vi "GetVolume.vi"(0 "reference in":refnum<class "MusicDevice.lvclass">, 5 "Error In":errorcluster) -> (14 "reference out":refnum<class "MusicDevice.lvclass">, 16 "Volume":u8 max=100, 19 "Error Out":errorcluster)   [LabVIEW 2024, in "MusicDevice.lvclass"]
uses:
  MusicDevice.lvclass
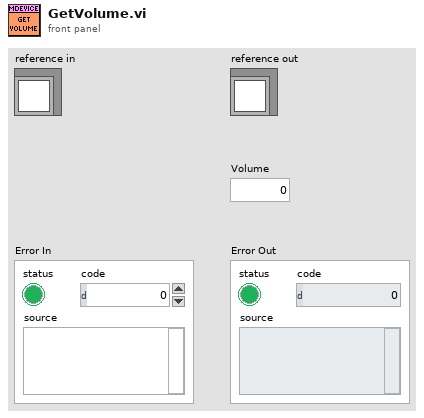
[diagram p1: front panel]
types:
  T1 = typedef "MusicDevice.lvclass/ObjectAttributes.ctl" = cluster{"State":bool, "Volume":u8}
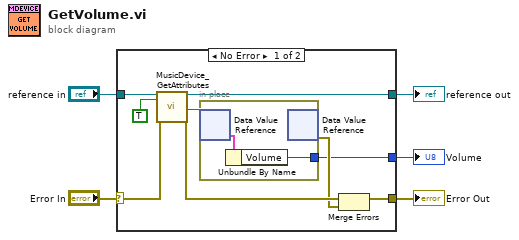
[diagram p0: block diagram]
diagram:
  n1 = case shown="No Error" "Error In" {
    selector: "Error In" -> [w14 w18]
    tunnel: [w12 w18] -> w4
    tunnel: [w9 w17] -> w2
    tunnel: "reference in" -> [w10 w17]
    tunnel: [w6 _] -> w1
    frame No Error {
      n2 = call "MusicDevice_GetAttributes.vi"("reference in"=w10, "OnlyGetDvrReference(False)"=TRUE, "Error In"=w14) -> ("reference out"=w9:refnum<class "MusicDevice.lvclass">, "DataRef"=w8:refnum<data-value>, "Error Out"=w13:errorcluster)  [unwired: 13 in, 1 out]
      n3 = in-place {
        in-place-border: [w16] -> w6
        n4 = in-place-dvr #1(w8) -> (w15:T1)  [unwired: 1 out]
        n5 = Unbundle By Name(w15) -> ("Volume"=w16:u8)
        n6 = in-place-dvr #1() -> (w11:errorcluster)  [unwired: 1 in, 1 out]
      }
      n7 = Merge Errors(w13, w11) -> (w12:errorcluster)
    }
    frame Error {
    }
  }
  "Error Out" <- w4
  "reference out" <- w2
  "Volume" <- w1
